vi "test_call_dll.vi"() -> ()   [LabVIEW 2020]
uses:
  gps_sim_sdr.dll
panel:
  out "error out":errorcluster
  out "return code":i32
  in  "param":string="-e brdc0010.22n -u circle.csv -d 10 -o filename"
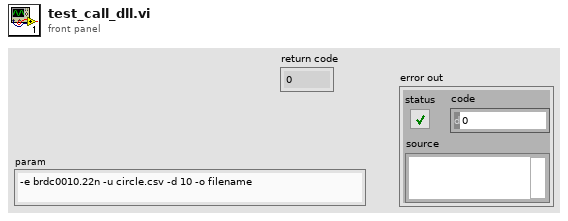
[diagram p1: front panel]
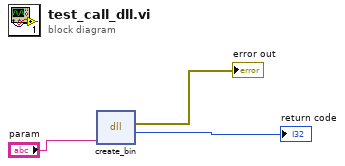
[diagram p0: block diagram]
diagram:
  n1 = dll-call lib="PTH2_abs CUsersduygaOneDriveデスクトップWORKSgps-sdr-sim-mastergps_sim_sdr.dll" fn="create_bin"("param"="param") -> (error out=→"error out":errorcluster, "return code"=→"return code":i32)  [unwired: 4 in, 1 out]
